vi "Create Evaluations.vi"(8 "error in (no error)":errorcluster, 11 "IEvaluation in":refnum<class "LTE_ACP.lvclass">) -> (0 "error out":errorcluster, 2 "Evaluations Out":T1[](array[typedef]) {"Low Limit" format="%#_13g"; "SI Scaling" items=["femto"=-15, "pico"=-12, "nano"=-9, "micro"=-6, "milli"=-3, "percent"=-2, ""=0, "kilo"=3, "mega"=6, "giga"=9, "tera"=12]}, 3 "IEvaluation out":refnum<class "LTE_ACP.lvclass">)   [LabVIEW 2016, in "SeqAuto Evaluations.lvlib" / "LTE_ACP.lvclass"]
uses:
  LTE_ACP.lvclass
  C:/Sequence Automation/Plugins/SeqAuto IEvaluation.lvlibp/SeqAuto IEvaluation.lvclass
  Plugins/TestStand API Tools (TSAT).lvlibp/Evaluation Actions/Includes/Controls/TSAT Evaluation.ctl
  Plugins/TestStand API Tools (TSAT).lvlibp/Evaluation Actions/Includes/Controls/TSAT Eval SI Unit Scaling.ctl
  Plugins/TestStand API Tools (TSAT).lvlibp/Evaluation Actions/Includes/Controls/TSAT Evaluation Type.ctl
  LTE_ACP.lvclass/LTE_ACP.ctl
  Private Methods/Read SA Pin.vi
  Plugins/SeqAuto IEvaluation.lvlibp/Read Measurement Name.vi
  Plugins/TestStand API Tools (TSAT).lvlibp/Evaluation Actions/TSAT Evaluation Actions.lvlib
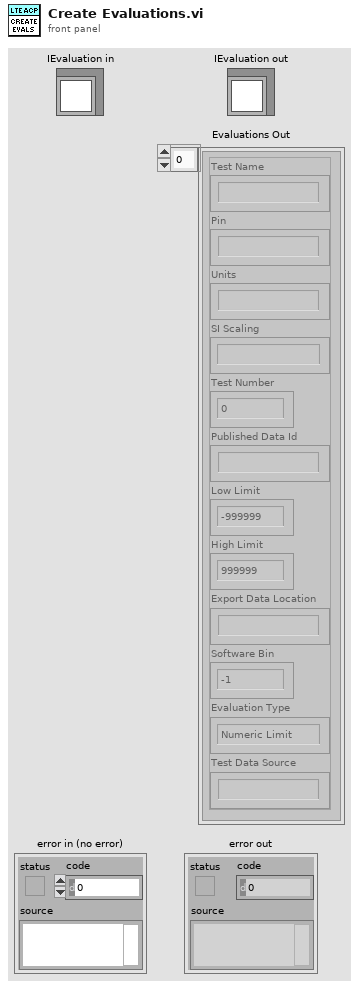
[diagram p1: front panel]
types:
  T1 = typedef "TestStand API Tools (TSAT).lvlibp/TSAT Evaluation Actions.lvlib/TSAT Evaluation.ctl" = cluster{"Test Name":string, "Pin":string, "Units":string, "SI Scaling":T2, "Test Number":i32, "Published Data Id":string, "Low Limit":dbl, "High Limit":dbl, "Export Data Location":string, "Software Bin":i64, "Evaluation Type":T3, "Test Data Source":string}
  T2 = typedef "TestStand API Tools (TSAT).lvlibp/TSAT Evaluation Actions.lvlib/TSAT Eval SI Unit Scaling.ctl" = i16
  T3 = typedef "TestStand API Tools (TSAT).lvlibp/TSAT Evaluation Actions.lvlib/TSAT Evaluation Type.ctl" = enum16{"Numeric Limit", "Pass/Fail", "None"}
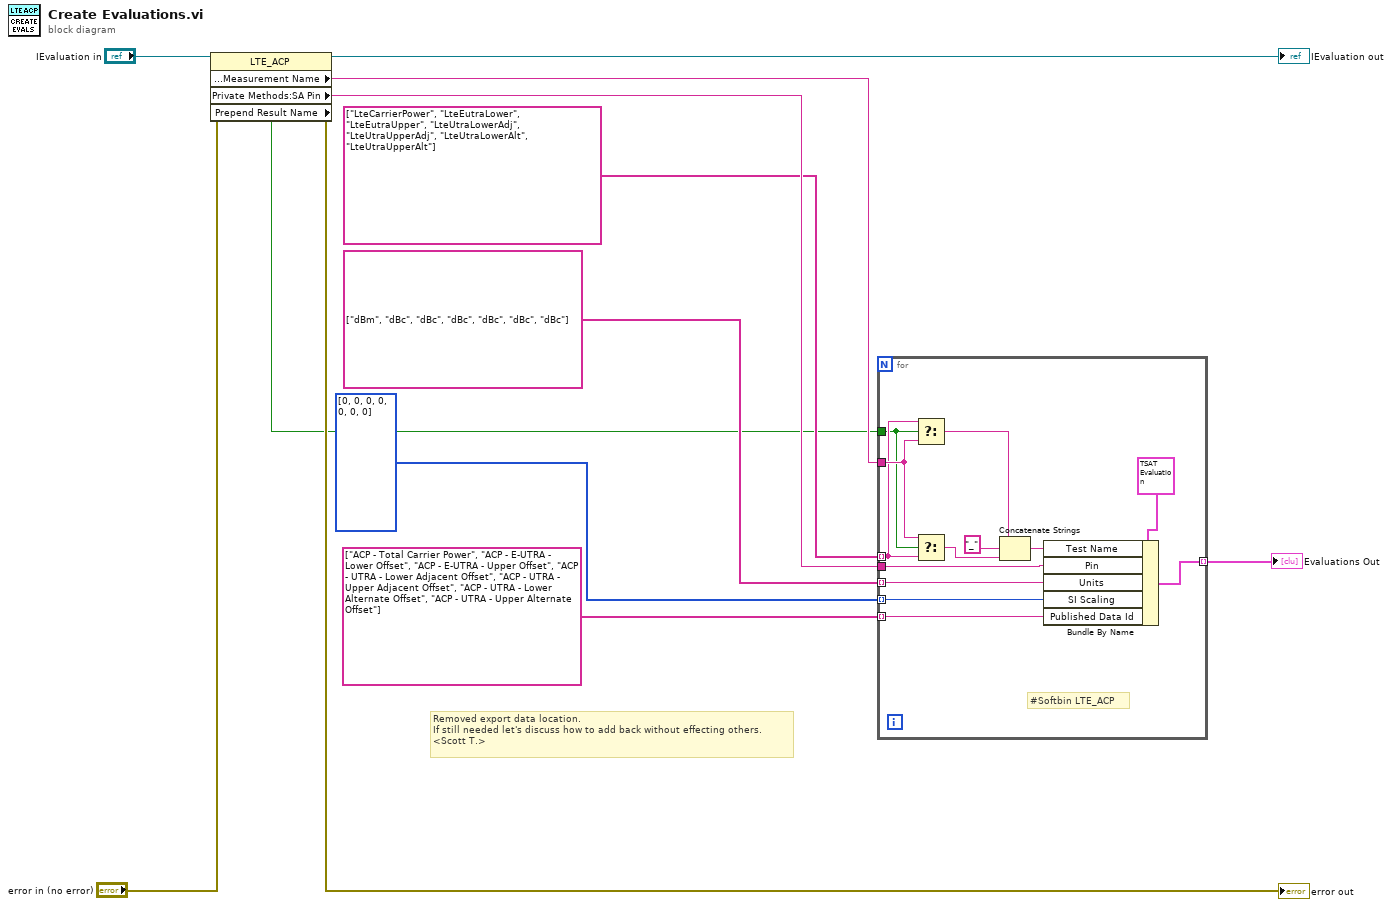
[diagram p0: block diagram]
diagram:
  w11 = T2[] [0, 0, 0, 0, 0, 0, 0] items=["femto"=-15, "pico"=-12, "nano"=-9, "micro"=-6, "milli"=-3, "percent"=-2, ""=0, "kilo"=3, "mega"=6, "giga"=9, "tera"=12]
  # "Removed export data location.\nIf still needed let's discuss how to add back without effecting others.\n<Scott T.>"
  n1 = property class="LTE_ACP"(reference="IEvaluation in", error in="error in (no error)") -> (reference out=→"IEvaluation out":refnum<class "LTE_ACP.lvclass">, error out=→"error out":errorcluster, "Protected Methods:Measurement Name"=w2:string, "Private Methods:SA Pin"=w9:string, "Prepend Result Name"=w1:bool)
  n2 = for {
    tunnel: [w24] -> w3 mode=indexing
    tunnel: string[] ["ACP - Total Carrier Power", "ACP - E-UTRA - Lower Offset", "ACP - E-UTRA - Upper Offset", "ACP - UTRA - Lower Adjacent Offset", "ACP - UTRA - Upper Adjacent Offset", "ACP - UTRA - Lower Alternate Offset", "ACP - UTRA - Upper Alternate Offset"] ("Array") -> [w23] mode=indexing
    tunnel: w11 -> [w22] mode=indexing
    tunnel: string[] ["dBm", "dBc", "dBc", "dBc", "dBc", "dBc", "dBc"] ("Array") -> [w21] mode=indexing
    tunnel: w9 -> [w20]
    tunnel: string[] ["LteCarrierPower", "LteEutraLower", "LteEutraUpper", "LteUtraLowerAdj", "LteUtraUpperAdj", "LteUtraLowerAlt", "LteUtraUpperAlt"] -> [w14] mode=indexing
    tunnel: w2 -> [w17]
    tunnel: w1 -> [w13]
    # "#Softbin LTE_ACP"
    n3 = Select(t=w14, s=w13, f=w17) -> (s? t:f=w16:string)
    n4 = Select(t=w17, s=w13, f=w14) -> (s? t:f=w15:string)
    n5 = Concatenate Strings(w16, "_" ("string"), w15) -> (w19:string)
    n6 = Bundle By Name(cluster=T1 {"Test Name"="", "Pin"="", "Units"="", "SI Scaling"=0, "Test Number"=0, "Published Data Id"="", "Low Limit"=-999999.0, "High Limit"=999999.0, "Export Data Location"="", "Software Bin"=-1, "Evaluation Type"=enum."Numeric Limit", "Test Data Source"=""} ("Evaluation"), "Test Name"=w19, "Pin"=w20, "Units"=w21, "SI Scaling"=w22, "Published Data Id"=w23) -> (w24:T1)
  }
  "Evaluations Out" <- w3
